vi "Get Neopixel RT DVR.vi"(8 "Error In":errorcluster, 11 "Display In":refnum<class "Neopixel - Host.lvclass">) -> (0 "Error Out":errorcluster, 2 "DVR":refnum<data-value>, 3 "Display Out":refnum<class "Neopixel - Host.lvclass">)   [LabVIEW 2021, in "Neopixel - Host.lvclass"]
uses:
  Neopixel - Host.lvclass
  Controls/Data.ctl
  Public/Controls/FPGA Reference.ctl
  Public/Controls/RGB Gains.ctl
  Neopixel - Host.lvclass/Neopixel - Host.ctl
  Display Utilities/Display Utilities.lvlib
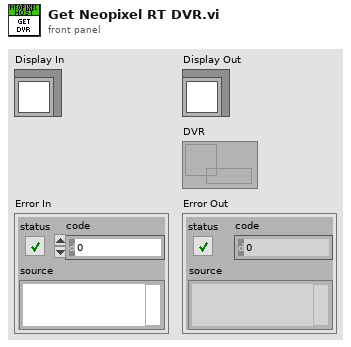
[diagram p1: front panel]
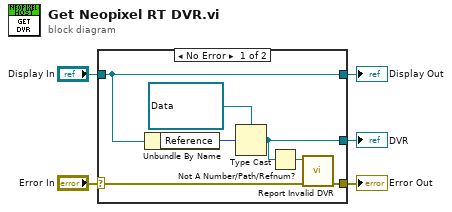
[diagram p0: block diagram]
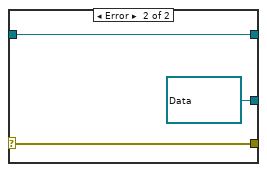
[diagram p2: hidden frame]
diagram:
  n1 = case shown="No Error" "Error In" {
    selector: "Error In" -> [w7 w15]
    tunnel: "Display In" -> [w11 w14]
    tunnel: [w6 w15] -> w3
    tunnel: [w11 w14] -> w2
    tunnel: [w9 refnum<data-value> refnum ("data value reference")] -> w1
    frame No Error {
      n2 = Unbundle By Name(w11) -> ("Reference"=w12:u64)
      n3 = Type Cast(type=refnum<data-value> refnum ("data value reference"), x=w12) -> (*(type *) &x=w9:refnum<data-value>)
      n4 = Not A Number/Path/Refnum?(number/path/refnum=w9) -> (NaN/Path/Refnum?=w8:bool)
      n5 = call "Report Invalid DVR.vi"("Error In"=w7, "Invalid DVR"=w8) -> ("Error Out"=w6:errorcluster)  [unwired: 9 in]
    }
    frame Error {
    }
  }
  "Display Out" <- w2
  "Error Out" <- w3
  "DVR" <- w1
